vi "Parse Arguments.vi"(8 "error in (no error)":errorcluster, 9 "Args":string[](array[string]), 10 "Folder":path, 11 "AddAction in":refnum<class "AddAction.lvclass">) -> (0 "error out":errorcluster, 3 "AddAction out":refnum<class "AddAction.lvclass">)   [LabVIEW 2020, in "GPackTools.lvlib" / "AddAction.lvclass"]
uses:
  AddAction.lvclass
  AddAction.lvclass/AddAction.ctl
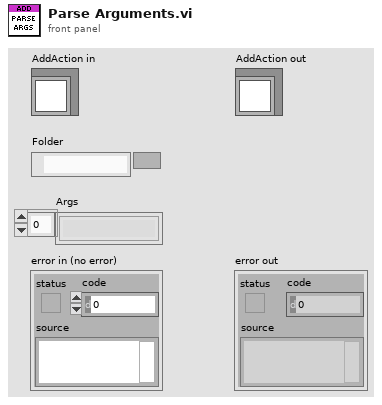
[diagram p1: front panel]
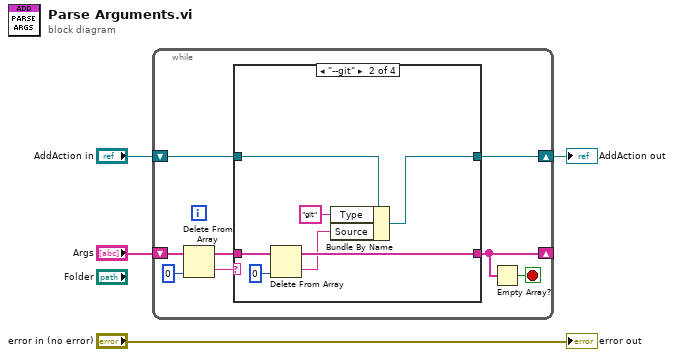
[diagram p0: block diagram]
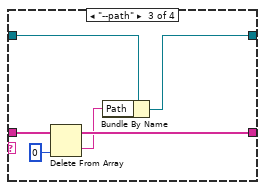
[diagram p3: hidden frame]
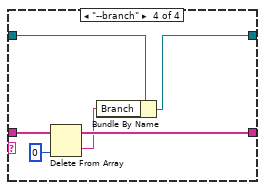
[diagram p4: hidden frame]
diagram:
  n1 = while {
    shift-right: [w5] -> w2
    shift-left: "AddAction in" -> [w6]
    shift-right: [w8] -> _
    shift-left: "Args" -> [w12]
    stop <- w7 stop-if-true
    n2 = Delete From Array(array=w12, index=0) -> (deleted portion=w10:string, array with subset deleted=w9:string[])  [unwired: 1 in]
    n3 = case shown="\"--git\"" w10 {
      tunnel: w9 -> [w14 w21 w27 w33]
      tunnel: [w14 w19 w25 w31] -> w8
      tunnel: w6 -> [w13 w20 w26 w32]
      tunnel: [w13 w17 w23 w29] -> w5
      frame Default {
      }
      frame "--git" {
        n4 = Delete From Array(array=w21, index=0) -> (deleted portion=w16:string, array with subset deleted=w19:string[])  [unwired: 1 in]
        n5 = Bundle By Name(cluster=w20, "Type"="git", "Source"=w16) -> (w17:refnum<class "AddAction.lvclass">)
      }
      frame "--path" {
        n6 = Delete From Array(array=w27, index=0) -> (deleted portion=w22:string, array with subset deleted=w25:string[])  [unwired: 1 in]
        n7 = Bundle By Name(cluster=w26, "Path"=w22) -> (w23:refnum<class "AddAction.lvclass">)
      }
      frame "--branch" {
        n8 = Delete From Array(array=w33, index=0) -> (deleted portion=w28:string, array with subset deleted=w31:string[])  [unwired: 1 in]
        n9 = Bundle By Name(cluster=w32, "Branch"=w28) -> (w29:refnum<class "AddAction.lvclass">)
      }
    }
    n10 = Empty Array?(array=w8) -> (empty?=w7:bool)
  }
  "AddAction out" <- w2
  "error out" <- "error in (no error)"
